vi "ClearBuffer.vi"(8 "错误输入（无错误）":errorcluster, 11 "设备类型":u32(ring)=3 items=["PCI5121"=1, "PCI9810"=2, "USBCAN1"=3, "USBCAN2"=4, "PCI9820"=5, "PCI5110"=7, "PC104CAN"=11, "CANETUDP"=12, "PCI9840B"=14, "PC104C2"=15, "PCI9820I"=16, "CANETTCP"=17, "PCIE9221"=24, "PCI5010U"=19, "USBCAN_E_U"=20, "USBCAN_2E_U"=21, "PCI5020U"=22]) -> (0 "错误输出":errorcluster, 2 "Result":bool, 3 "DeviceType":u32)   [LabVIEW 2013]
uses:
  ControlCAN.dll
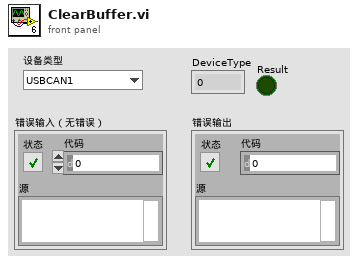
[diagram p1: front panel]
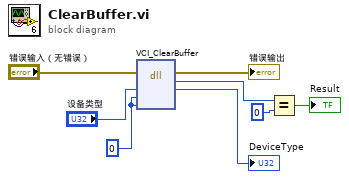
[diagram p0: block diagram]
diagram:
  w8 = u32 0 ("CANInd")
  n1 = dll-call lib="PTH1abs Déè¯å¡å°å¡å°æµè¯æºå¡å°CS10æåæµè¯ç¨åº\nSourcecodeCS10 TestSystemInstrumentDriversZLGCAN_labviewControlCAN.dll" fn="VCI_ClearBuffer"(error in="错误输入（无错误）", "DeviceType"="设备类型", "DeviceInd"=w8, "CANInd"=w8) -> (error out=→"错误输出":errorcluster, w3:u32, "DeviceType"=→"DeviceType":u32)  [unwired: 4 in, 1 out]
  n2 = Equal?(x=w3, y=u32 0) -> (x = y?=→"Result":bool)
